vi "OCR_Detect Color Set change.vi"(8 "New Color Set":T1, 11 "Previous Color Set":T1) -> (3 "Color Change Out":bool)   [LabVIEW 2009]
uses:
  Controls/Cluster/Cluster_Text Color Set.ctl
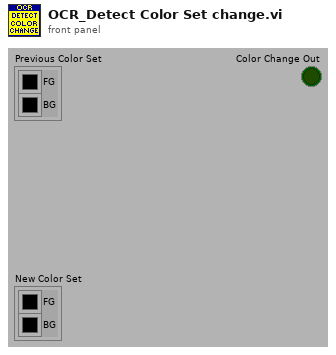
[diagram p1: front panel]
types:
  T1 = typedef "Cluster_Text Color Set.ctl" = cluster{"BG":u32, "FG":u32}
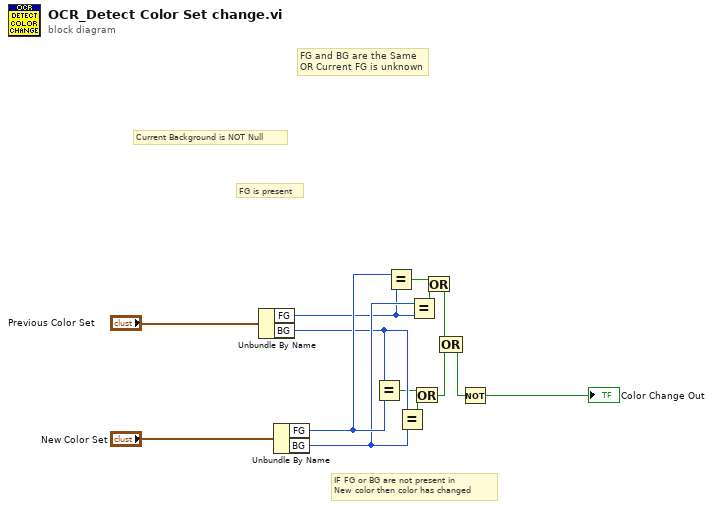
[diagram p0: block diagram]
diagram:
  # "IF FG or BG are not present in \nNew color then color has changed"
  # "FG is present"
  # "Current Background is NOT Null"
  # "FG and BG are the Same\nOR Current FG is unknown"
  n1 = Unbundle By Name("Previous Color Set") -> ("FG"=w8:u32, "BG"=w9:u32)
  n2 = Unbundle By Name("New Color Set") -> ("FG"=w13:u32, "BG"=w10:u32)
  n3 = Equal?(x=w9, y=w13) -> (x = y?=w7:bool)
  n4 = Equal?(x=w13, y=w8) -> (x = y?=w5:bool)
  n5 = Equal?(x=w9, y=w10) -> (x = y?=w6:bool)
  n6 = Equal?(x=w10, y=w8) -> (x = y?=w4:bool)
  n7 = Or(x=w7, y=w6) -> (x .or. y?=w2:bool)
  n8 = Or(x=w5, y=w4) -> (x .or. y?=w3:bool)
  n9 = Compound Arithmetic op=OR(w3, w2) -> (w1:bool)
  n10 = Not(x=w1) -> (.not. x?=→"Color Change Out":bool)
